vi "DC Motor Main.vi"() -> ()   [LabVIEW 2021]
uses:
  DC Motor.lvclass
  Communication/Comm/Comm.lvclass
  Communication/Serial/Serial.lvclass
  Communication/Wifi/Wifi.lvclass
panel:
  in  "Duty Cycle":dbl
  out "Echo":string
  in  "Time on (ms)":dbl
  in  "Turn Motor on":bool
  in  "Stop":bool
  in  "Motor Signal":dbl(graph)
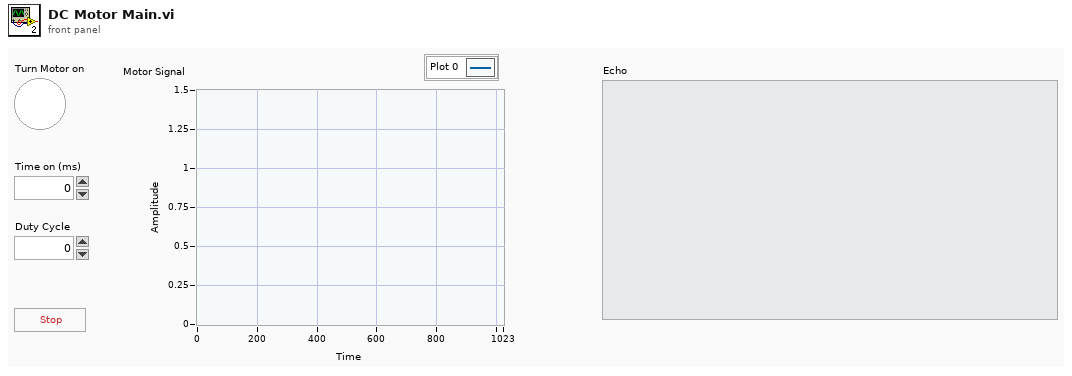
[diagram p1: front panel]
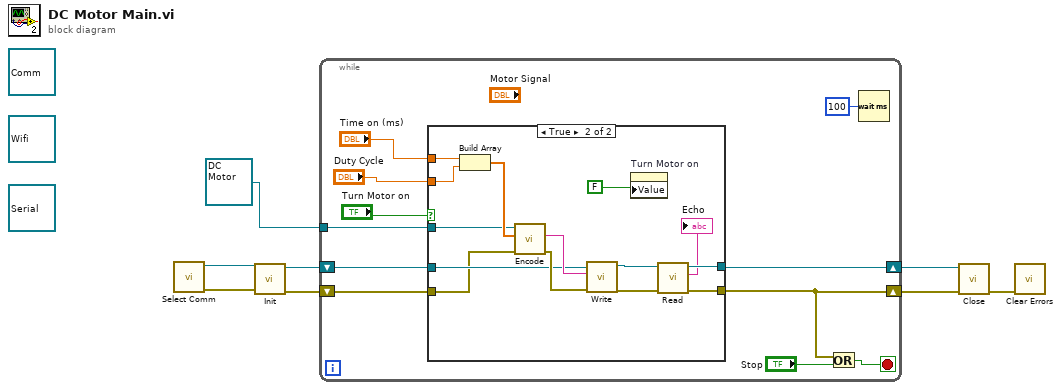
[diagram p0: block diagram]
diagram:
  (unwired) refnum<class "Wifi.lvclass"> refnum ("Wifi.lvclass")
  (unwired) refnum<class "Serial.lvclass"> refnum ("Serial.lvclass")
  (unwired) refnum<class "Comm.lvclass"> refnum ("Comm in")
  n1 = call "Select Comm.vi"() -> ("error out"=w4:errorcluster, "Comm.lvclass"=w5:refnum<class "Comm.lvclass">)  [unwired: 10 in]
  n2 = call-dynamic "Init.vi"("error in (no error)"=w4, "Comm in"=w5) -> ("error out"=w8:errorcluster, "Comm out"=w6:refnum<class "Comm.lvclass">)  [unwired: 8 in]
  n3 = while {
    shift-right: [w14] -> w3
    shift-left: w8 -> [w11]
    shift-right: [w13] -> w7
    shift-left: w6 -> [w12]
    tunnel: refnum<class "DC Motor.lvclass"> refnum ("DC Motor.lvclass") -> [w9]
    stop <- w15 stop-if-true
    n4 = case shown="True" "Turn Motor on" {
      tunnel: "Time on (ms)" -> [_ w25]
      tunnel: [w20 w30] -> w14
      tunnel: [w21 w29] -> w13
      tunnel: w12 -> [w21 w28]
      tunnel: w11 -> [w20 w27]
      tunnel: "Duty Cycle" -> [_ w24]
      tunnel: w9 -> [_ w22]
      frame False {
      }
      frame True {
        n5 = Build Array(w25, w24) -> (w23:dbl[])
        n6 = call-dynamic "Encode.vi"("error in (no error)"=w27, "Data"=w23, "DC Motor in"=w22) -> ("error out"=w35:errorcluster, "Message"=w34:string)  [unwired: 6 in, 1 out]
        n7 = call-dynamic "Write.vi"("error in (no error)"=w35, "Message"=w34, "Comm in"=w28) -> ("error out"=w32:errorcluster, "Comm out"=w31:refnum<class "Comm.lvclass">)  [unwired: 7 in]
        n8 = property on="Turn Motor on" class="Bool (strict)"("Value"=FALSE ("Turn Motor on")) -> ()  [unwired: 2 in, 2 out]
        n9 = call-dynamic "Read.vi"("error in (no error)"=w32, "Comm in"=w31) -> ("error out"=w30:errorcluster, "Message"=→"Echo":string, "Comm out"=w29:refnum<class "Comm.lvclass">)  [unwired: 7 in]
      }
    }
    n10 = Or(x=w14, y="Stop") -> (x .or. y?=w15:bool)
    n11 = Wait (ms)(milliseconds to wait=u32 100) -> ()  [unwired: 1 out]
  }
  n12 = call-dynamic "Close.vi"("error in (no error)"=w3, "Comm in"=w7) -> ("error out"=w2:errorcluster)  [unwired: 8 in, 1 out]
  n13 = call <vilib>:"Clear Errors.vi"("error in (no error)"=w2) -> ()  [unwired: 5 in, 2 out]
